vi "Get ControlRef from ClassItem.vi"(8 "error in (no error)":errorcluster, 10 "item name":string, 11 "class in":refnum<vi>) -> (0 "error out":errorcluster, 1 "control":refnum<vi>, 2 "VI ref out":refnum<vi>, 3 "class out":refnum<vi>, 4 "found":bool)   [LabVIEW 2019, in "gRPC Template Creation Utility.lvlib"]
uses:
  gRPC Template Creation Utility.lvlib
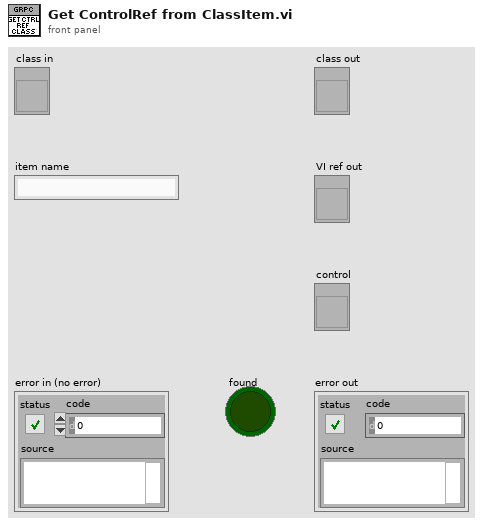
[diagram p1: front panel]
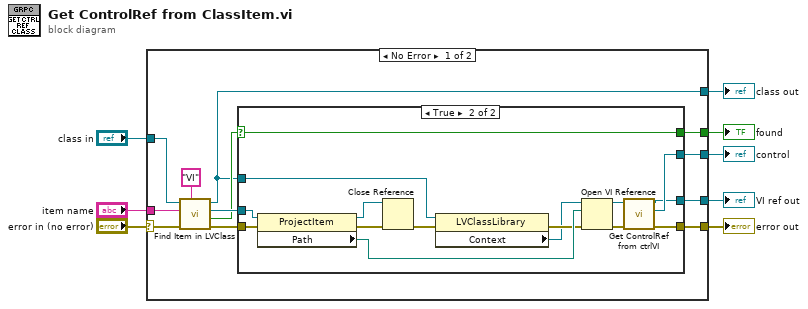
[diagram p0: block diagram]
diagram:
  n1 = case shown="No Error" "error in (no error)" {
    selector: "error in (no error)" -> [w13 w38]
    tunnel: [w20 _] -> w8
    tunnel: "class in" -> [w17 w39]
    tunnel: "item name" -> [w15 _]
    tunnel: [w10 w39] -> w5
    tunnel: [w14 w38] -> w4
    tunnel: [w11 _] -> w2
    tunnel: [w9 _] -> w1
    frame No Error {
      n2 = call "Find Item in LVClass.vi"("Item Type"="VI", "error in (no error)"=w13, "Item Name"=w15, "Class Item in"=w17) -> ("error out"=w19:errorcluster, "Found?"=w12:bool, "Project Item (Class Item)"=w18:refnum<vi>, "Class Item out"=w10:refnum<vi>)  [unwired: 4 in]
      n3 = case shown="True" w12 {
        selector: w12 -> [w21 w31]
        tunnel: [_ w36] -> w20
        tunnel: w19 -> [w22 w34]
        tunnel: w18 -> [_ w33]
        tunnel: [w22 w24] -> w14
        tunnel: [w21 w31] -> w11
        tunnel: w10 -> [_ w30]
        tunnel: [_ w23] -> w9
        frame False {
        }
        frame True {
          n4 = property class="ProjectItem"(reference=w33, error in=w34) -> (reference out=w25:refnum<vi>, error out=w27:errorcluster, "Path"=w32:path)
          n5 = Close Reference(reference=w25, error in (no error)=w27) -> (error out=w26:errorcluster)
          n6 = property class="LVClassLibrary"(reference=w30, error in=w26) -> (error out=w29:errorcluster, "Context"=w28:refnum<vi>)  [unwired: 1 out]
          n7 = Open VI Reference(application reference (local)=w28, vi path=w32, error in (no error)=w29) -> (vi reference=w35:refnum<vi>, error out=w37:errorcluster)  [unwired: 3 in]
          n8 = call "Get ControlRef from ctrlVI.vi"("error in (no error)"=w37, "VI ref in"=w35) -> ("error out"=w24:errorcluster, "Control ref out"=w36:refnum<vi>, "VI ref out"=w23:refnum<vi>)  [unwired: 7 in]
        }
      }
    }
    frame Error {
    }
  }
  "control" <- w8
  "class out" <- w5
  "error out" <- w4
  "found" <- w2
  "VI ref out" <- w1
